vi "AB_Get_VI_Scope.vi"(8 "error in (no error)":errorcluster, 11 "vi reference":refnum<vi>) -> (0 "error out":errorcluster, 2 "Source Scope":T1(ring), 3 "dup vi reference":refnum<vi>)   [LabVIEW 2020]
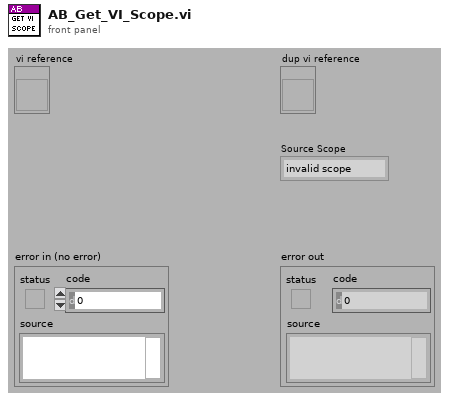
[diagram p1: front panel]
types:
  T1 = enum32{"invalid scope", "public", "private", "protected", "community"}
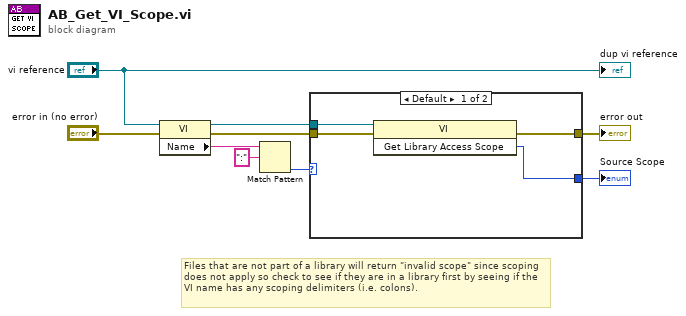
[diagram p0: block diagram]
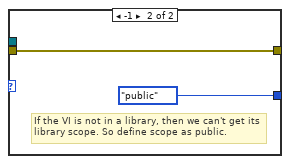
[diagram p2: hidden frame]
diagram:
  # "Files that are not part of a library will return \"invalid scope\" since scoping does not apply so check to see if they are in a library first by seeing if the VI name has any scoping delimiters (i.e. colons)."
  n1 = property class="VI"(reference="vi reference", error in="error in (no error)") -> (reference out=w6:refnum<vi>, error out=w2:errorcluster, "Name"=w7:string)
  n2 = Match Pattern(string=w7, regular expression=":" ("search string/char (-)")) -> (offset past match=w8:i32)  [unwired: 4 out]
  n3 = case shown="Default" w8 {
    tunnel: [w10 T1."public" ("Source Scope")] -> w3
    tunnel: w6 -> [w13 _]
    tunnel: w2 -> [w12 w14]
    tunnel: [w11 w14] -> w1
    frame Default {
      n4 = invoke class="VI" method="Get Library Access Scope"(reference=w13, error in=w12) -> (error out=w11:errorcluster, "Get Library Access Scope"=w10:T1)  [unwired: 1 in, 1 out]
    }
    frame -1 {
      # "If the VI is not in a library, then we can't get its library scope. So define scope as public."
    }
  }
  "error out" <- w1
  "Source Scope" <- w3
  "dup vi reference" <- "vi reference"
